vi "FGV variant.vi"(9 "Response to save":string, 10 "Command":string, 11 "Functions":T1(ring)) -> (2 "Response retrieved":string, 3 "Variant":variant)   [LabVIEW 2020, in "Simulado.lvclass"]
uses:
  Simulado.lvclass
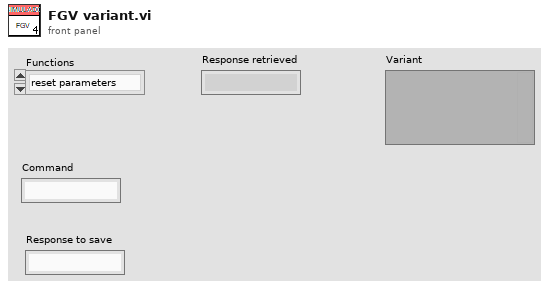
[diagram p1: front panel]
types:
  T1 = enum16{"reset parameters", "Get parameters", "Set parameter"}
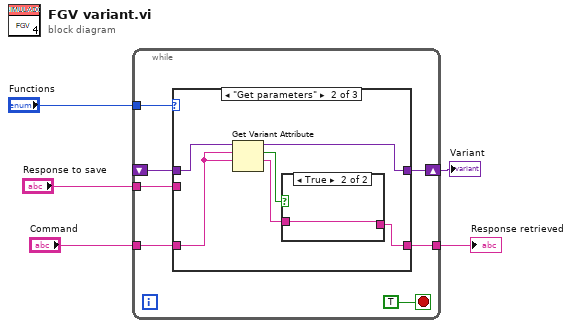
[diagram p0: block diagram]
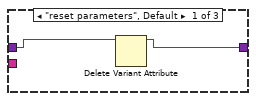
[diagram p2: hidden frame]
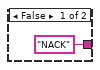
[diagram p3: hidden frame]
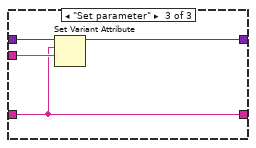
[diagram p4: hidden frame]
diagram:
  n1 = while {
    tunnel: "Functions" -> [w12]
    tunnel: "Command" -> [w11]
    tunnel: [w10] -> w4
    shift-right: [w8] -> w3
    shift-left: _ -> [w9]
    tunnel: "Response to save" -> [w7]
    stop <- TRUE stop-if-true
    n2 = case shown="\"Get parameters\"" w12 {
      tunnel: [_ w16 w23] -> w10
      tunnel: w11 -> [_ w18 w23]
      tunnel: w9 -> [w14 w19 w26]
      tunnel: [w13 w20 w25] -> w8
      tunnel: w7 -> [_ _ w24]
      frame "reset parameters", Default {
        n3 = Delete Variant Attribute(7:w14) -> (3:w13:variant)  [unwired: 2 in, 2 out]
      }
      frame "Get parameters" {
        n4 = Get Variant Attribute(Variant=w19, name=w18, default value (empty Variant)=w18) -> (duplicate Variant=w20:variant, found=w15:bool, value=w17:string)  [unwired: 1 in, 1 out]
        n5 = case shown="True" w15 {
          tunnel: w17 -> [_ w22]
          tunnel: ["NACK" ("Command") w22] -> w16
          frame False {
          }
          frame True {
          }
        }
      }
      frame "Set parameter" {
        n6 = Set Variant Attribute(Variant=w26, name=w23, value=w24) -> (Variant out=w25:variant)  [unwired: 1 in, 2 out]
      }
    }
  }
  "Response retrieved" <- w4
  "Variant" <- w3
